vi "__FilterSet_SelectModeChange.vi"(4 "EIDRef 2":refnum<vi>[](array[refnum]), 6 "IDRef 2":refnum<vi>[](array[refnum]), 7 "Mode":T2(ring), 8 "error in (no error)":errorcluster, 9 "EIDRef":refnum<vi>[](array[refnum]), 10 "IDRef":refnum<vi>[](array[refnum]), 11 "CtrlRef":T1) -> (0 "error out":errorcluster)   [LabVIEW 2011]
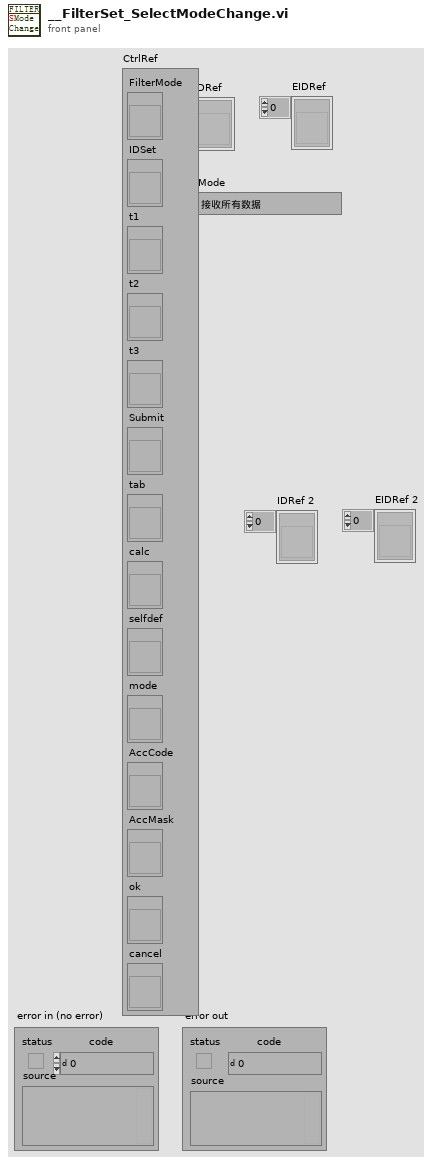
[diagram p1: front panel]
types:
  T1 = cluster{"FilterMode":refnum<vi>, "IDSet":refnum<vi>, "t1":refnum<vi>, "t2":refnum<vi>, "t3":refnum<vi>, "Submit":refnum<vi>, "tab":refnum<vi>, "calc":refnum<vi>, "selfdef":refnum<vi>, "mode":refnum<vi>, "AccCode":refnum<vi>, "AccMask":refnum<vi>, "ok":refnum<vi>, "cancel":refnum<vi>}
  T2 = enum16{"接收所有数据", "标准帧滤波（设定接收单个ID）", "扩展帧滤波（设定接收单个ID）", "标准帧滤波（仅ID，自由设定）", "扩展帧滤波（仅ID，自由设定）"}
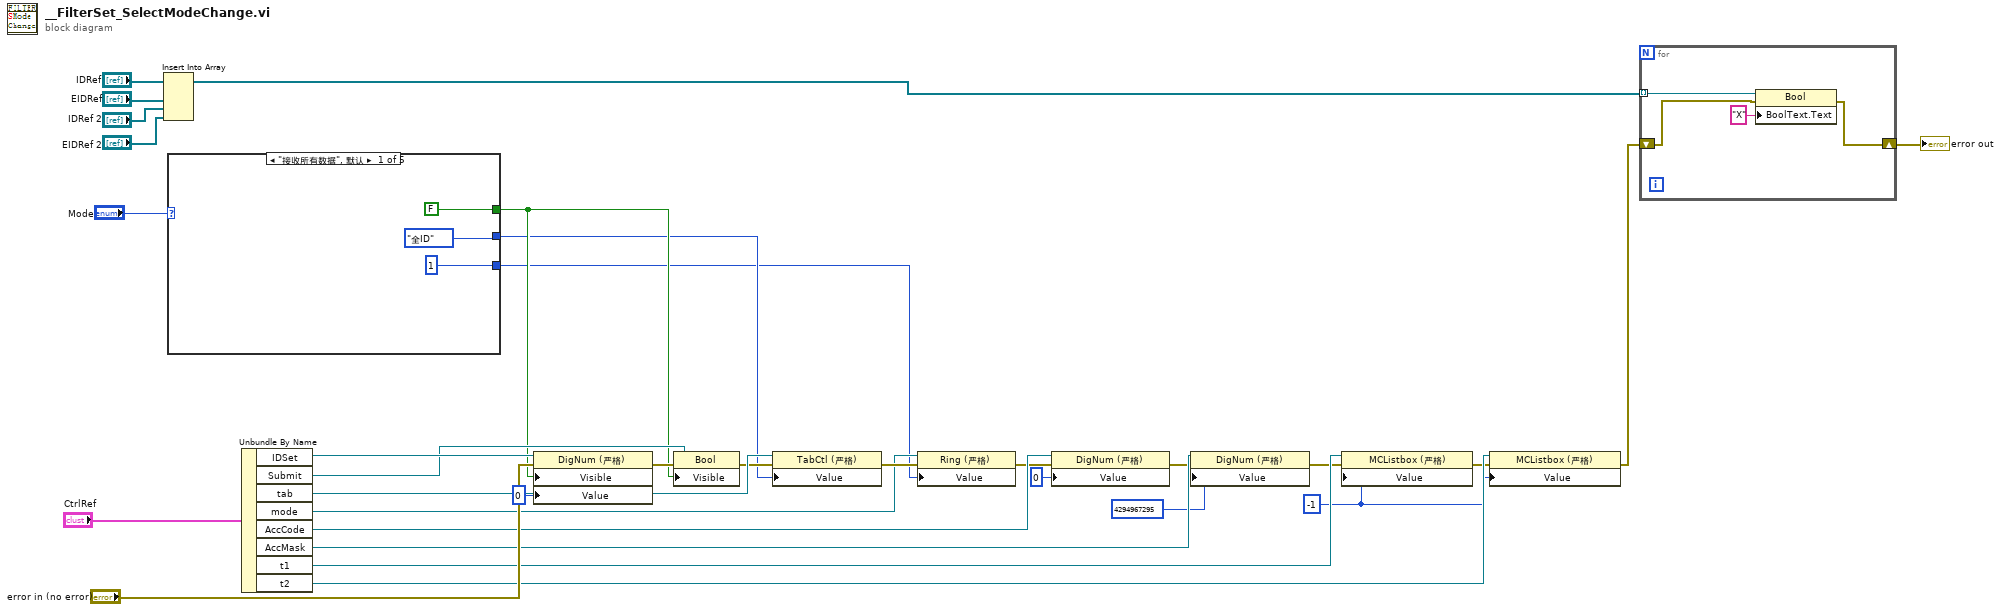
[diagram p0: block diagram]
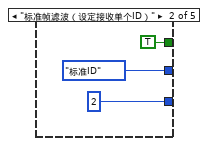
[diagram p2: hidden frame]
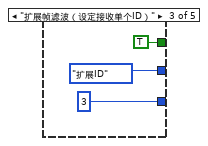
[diagram p3: hidden frame]
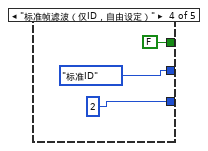
[diagram p4: hidden frame]
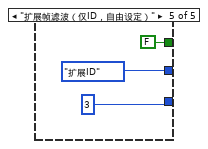
[diagram p5: hidden frame]
diagram:
  w5 = -1 ("值")
  n1 = Insert Into Array(array="IDRef", new element #1="EIDRef", new element #2="IDRef 2", new element #3="EIDRef 2") -> (w12:refnum<vi>[])  [unwired: 1 in]
  n2 = case shown="\"接收所有数据\", 默认" "Mode" {
    tunnel: [FALSE TRUE TRUE FALSE FALSE] -> w27
    tunnel: [enum32{"标准ID", "扩展ID", "全ID"}."全ID" ("tab") enum32{"标准ID", "扩展ID", "全ID"}."标准ID" ("tab") enum32{"标准ID", "扩展ID", "全ID"}."扩展ID" ("tab") enum32{"标准ID", "扩展ID", "全ID"}."标准ID" ("tab") enum32{"标准ID", "扩展ID", "全ID"}."扩展ID" ("tab")] -> w24
    tunnel: [u8 1 ("值") u8 2 ("值") u8 3 ("值") u8 2 ("值") u8 3 ("值")] -> w21
    frame "接收所有数据", Default {
    }
    frame "标准帧滤波（设定接收单个ID）" {
    }
    frame "扩展帧滤波（设定接收单个ID）" {
    }
    frame "标准帧滤波（仅ID，自由设定）" {
    }
    frame "扩展帧滤波（仅ID，自由设定）" {
    }
  }
  n3 = Unbundle By Name("CtrlRef") -> ("IDSet"=w31:refnum<vi>, "Submit"=w29:refnum<vi>, "tab"=w26:refnum<vi>, "mode"=w22:refnum<vi>, "AccCode"=w20:refnum<vi>, "AccMask"=w19:refnum<vi>, "t1"=w9:refnum<vi>, "t2"=w8:refnum<vi>)
  n4 = property class="DigNum (严格)"(reference=w31, error in="error in (no error)", "Visible"=w27, "Value"=u32 0 ("值")) -> (error out=w28:errorcluster)  [unwired: 1 out]
  n5 = property class="Bool"(reference=w29, error in=w28, "Visible"=w27) -> (error out=w25:errorcluster)  [unwired: 1 out]
  n6 = property class="TabCtl (严格)"(reference=w26, error in=w25, "Value"=w24) -> (error out=w23:errorcluster)  [unwired: 1 out]
  n7 = property class="Ring (严格)"(reference=w22, error in=w23, "Value"=w21) -> (error out=w18:errorcluster)  [unwired: 1 out]
  n8 = property class="DigNum (严格)"(reference=w20, error in=w18, "Value"=u32 0 ("值")) -> (error out=w17:errorcluster)  [unwired: 1 out]
  n9 = property class="DigNum (严格)"(reference=w19, error in=w17, "Value"=u32 4294967295 ("值")) -> (error out=w6:errorcluster)  [unwired: 1 out]
  n10 = property class="MCListbox (严格)"(reference=w9, error in=w6, "Value"=w5) -> (error out=w7:errorcluster)  [unwired: 1 out]
  n11 = property class="MCListbox (严格)"(reference=w8, error in=w7, "Value"=w5) -> (error out=w4:errorcluster)  [unwired: 1 out]
  n12 = for {
    tunnel: w12 -> [w51] mode=indexing
    shift-right: [w48] -> w11
    shift-left: w4 -> [w49]
    n13 = property class="Bool"(reference=w51, error in=w49, "BoolText.Text"="X" ("布尔文本.文本")) -> (error out=w48:errorcluster)  [unwired: 1 out]
  }
  "error out" <- w11
